vi "test clear jkism string queue in API1.vi"() -> ()   [LabVIEW 2017]
uses:
  user.lib/_NEVSTOP/Communicable State Machine(CSM)/AdvanceAPI/CSM - Revert Arguments-Safe String.vi
  user.lib/_NEVSTOP/Communicable State Machine(CSM)/AdvanceAPI/CSM - Make String Arguments Safe.vi
  user.lib/_NEVSTOP/Communicable State Machine(CSM)/AdvanceAPI/CSM - Break Down Multiple States String.vi
  user.lib/_NEVSTOP/Communicable State Machine(CSM)/AdvanceAPI/CSM - Compact Multiple States.vi
  user.lib/_NEVSTOP/Communicable State Machine(CSM)/AdvanceAPI/CSM - Keywords.vi
  user.lib/_NEVSTOP/Communicable State Machine(CSM)/_Shared/Trim Single-line Text.vi
  user.lib/_NEVSTOP/Communicable State Machine(CSM)/Communicable State Machine.lvlib
panel:
  in  "API: API1 ->| CSM-Module":bool
  in  "API: API1 -@ CSM-Module":bool
  in  "API: API1 -> CSM-Module":bool
  out "State History 2":string
  out "Error Occurred":errorcluster
  out "State History":string
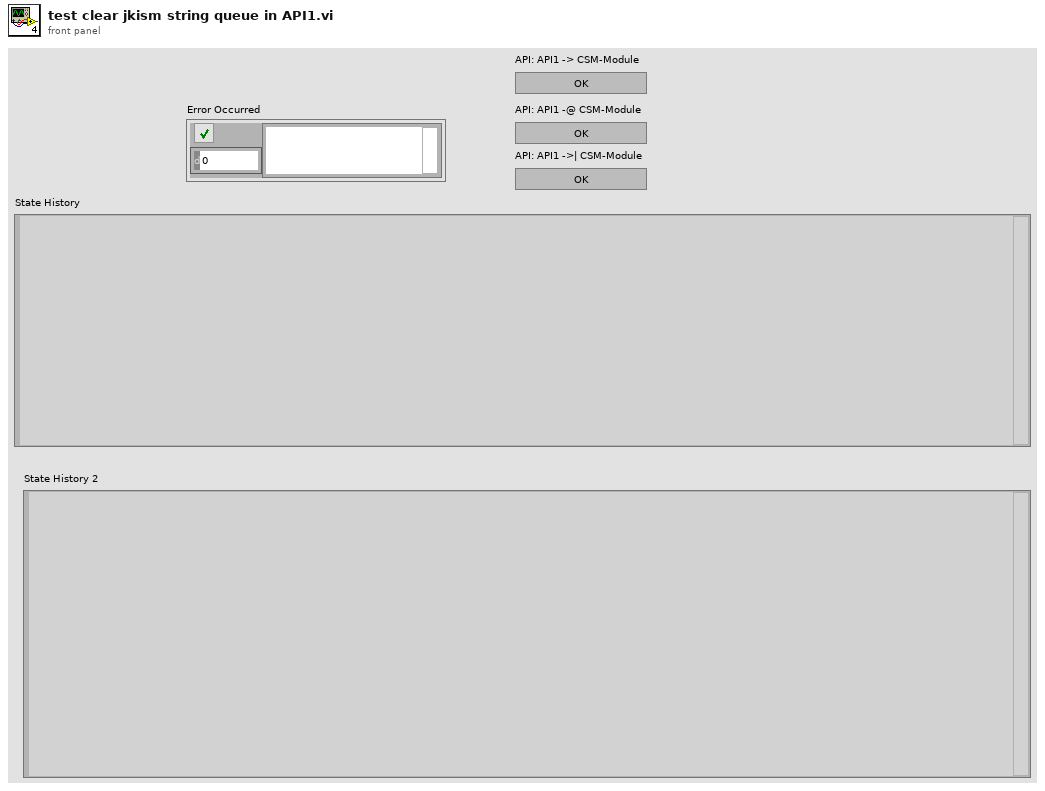
[diagram p1: front panel]
types:
  T1 = enum32{"Invalid", "Standard", "Closed", "Hidden", "Minimized", "Maximized"}
  T2 = enum32{"invalid app kind", "Development System", "Run Time System", "Student Edition", "Embedded LabVIEW", "Evaluation", "Custom"}
  T3 = typedef "Communicable State Machine.lvlib/_CSM_Response Source Message.ctl" = cluster{"‘State":string, "’Arguments":string, "’Error":errorcluster}
  T4 = cluster{"Current VI Reference":refnum<vi>, "Close Panel on Exit?":bool}
  T5 = cluster{"Core":cluster{"Current VI Reference":refnum<vi>, "Close Panel on Exit?":bool}, "Your Boolean data":bool, "Your string data":string}
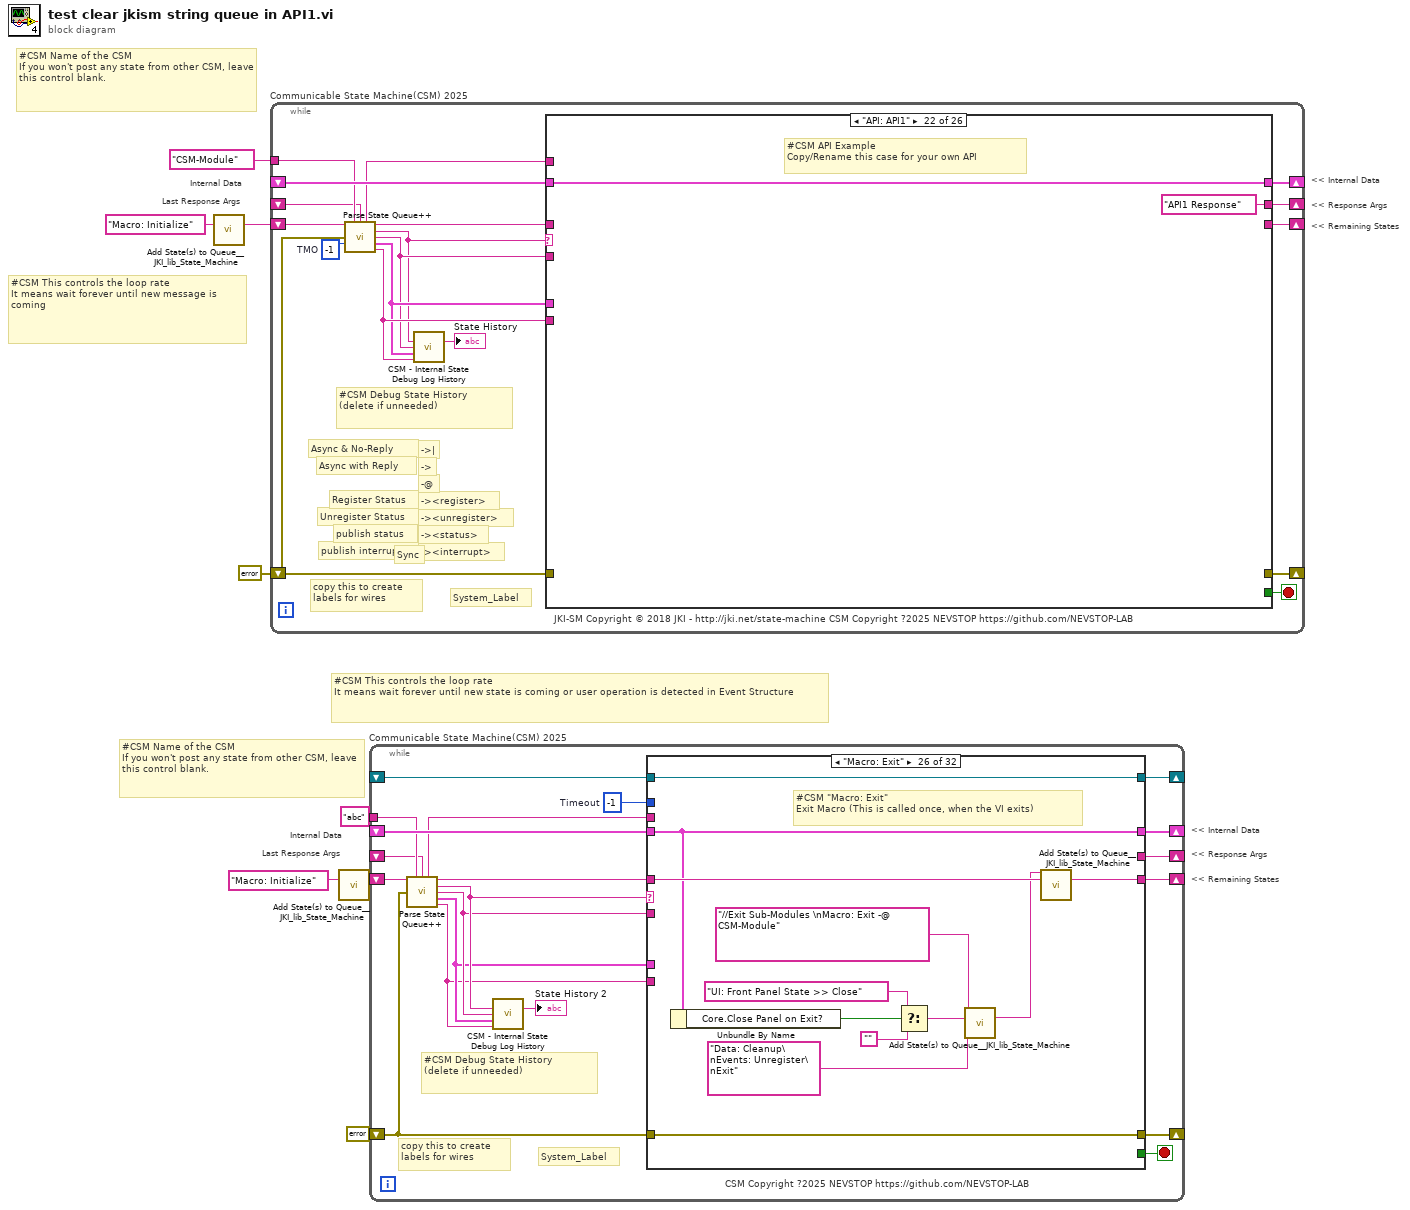
[diagram p0: block diagram]
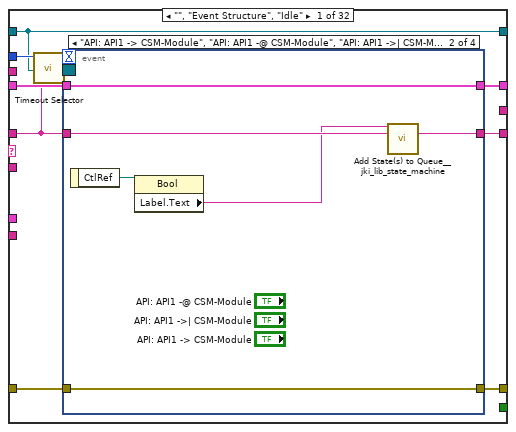
[diagram p2: hidden frame]
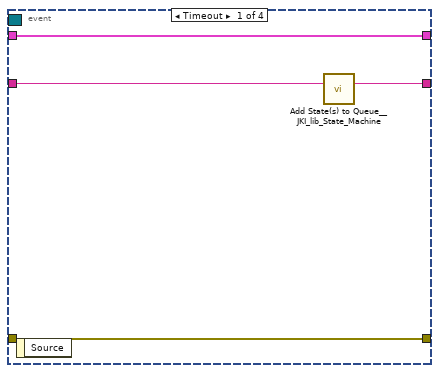
[diagram p3: hidden frame]
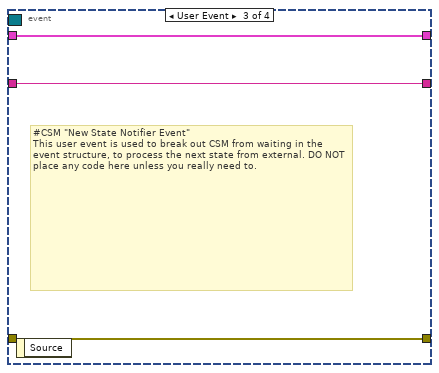
[diagram p4: hidden frame]
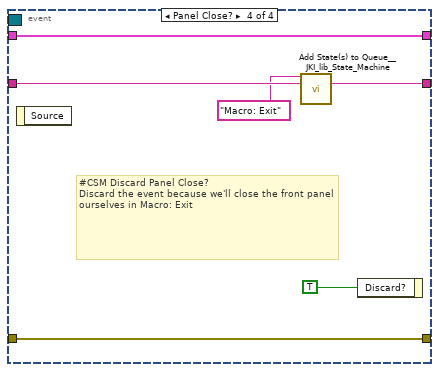
[diagram p5: hidden frame]
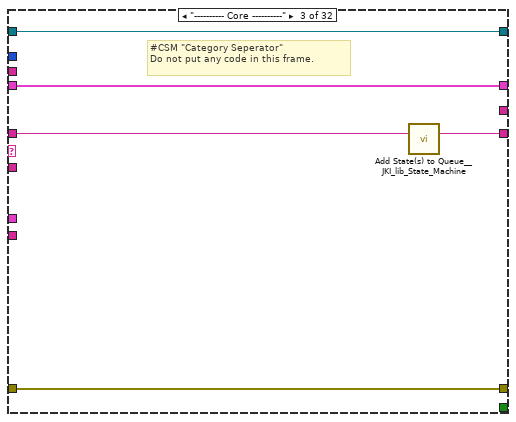
[diagram p7: hidden frame]
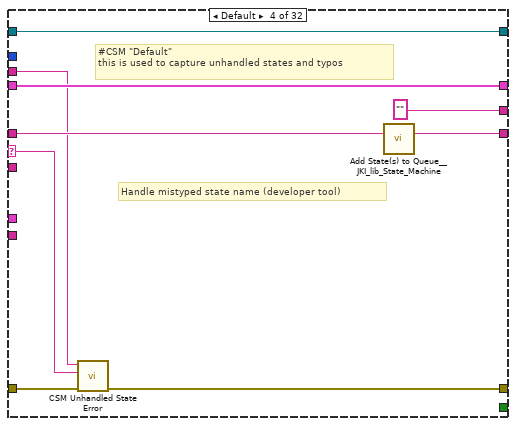
[diagram p8: hidden frame]
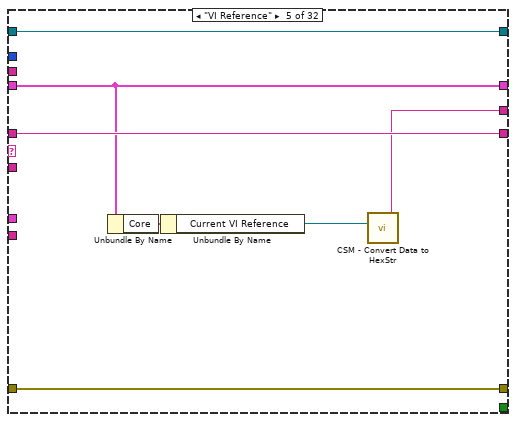
[diagram p9: hidden frame]
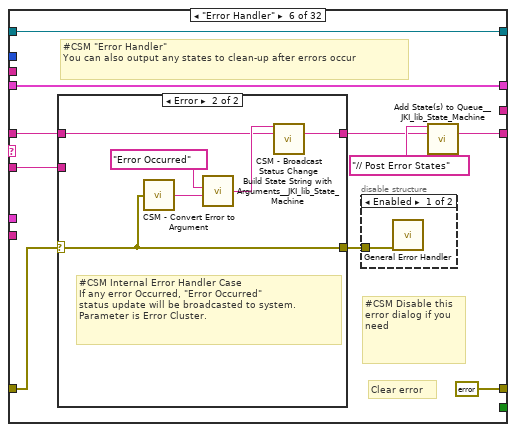
[diagram p10: hidden frame]
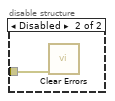
[diagram p11: hidden frame]
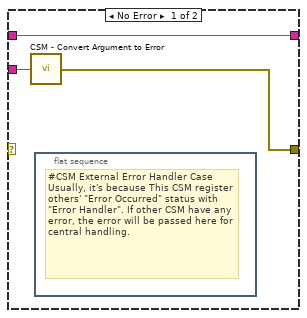
[diagram p12: hidden frame]
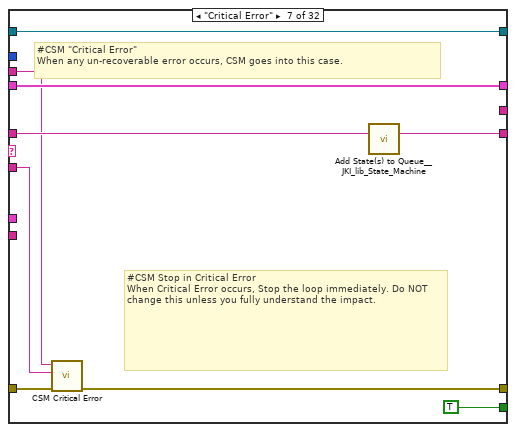
[diagram p13: hidden frame]
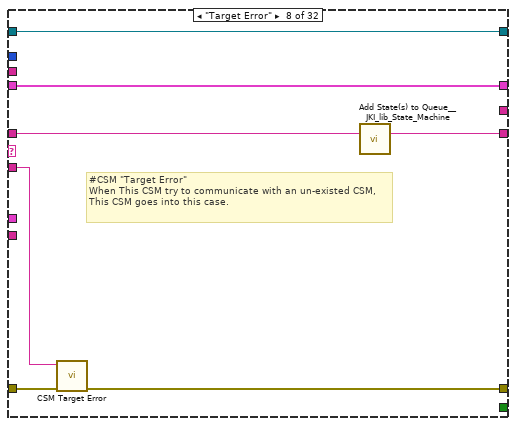
[diagram p14: hidden frame]
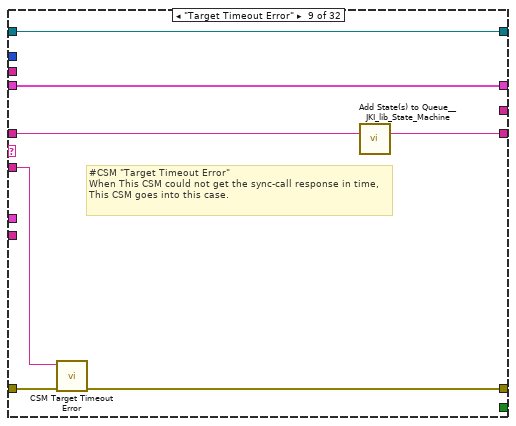
[diagram p15: hidden frame]
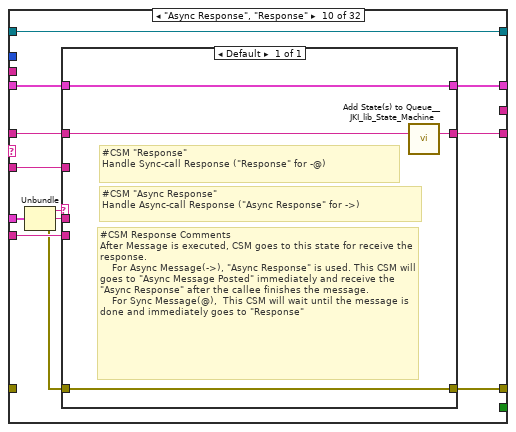
[diagram p16: hidden frame]
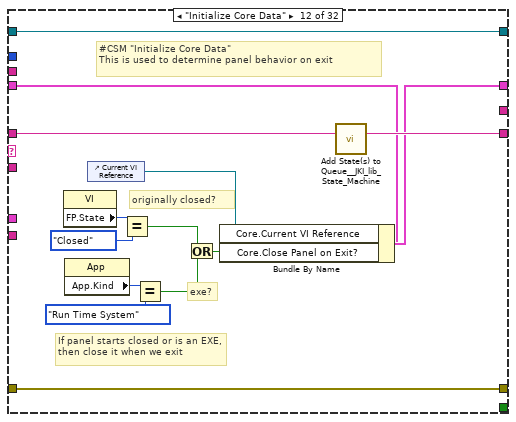
[diagram p18: hidden frame]
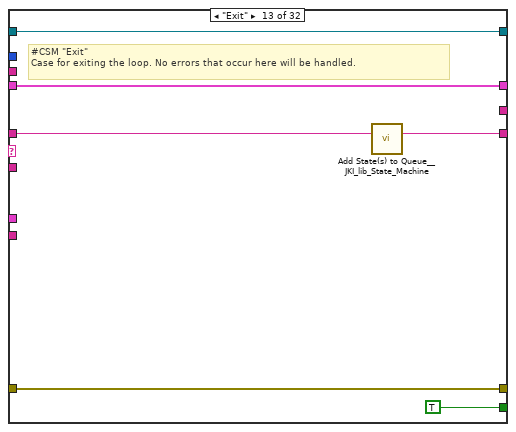
[diagram p19: hidden frame]
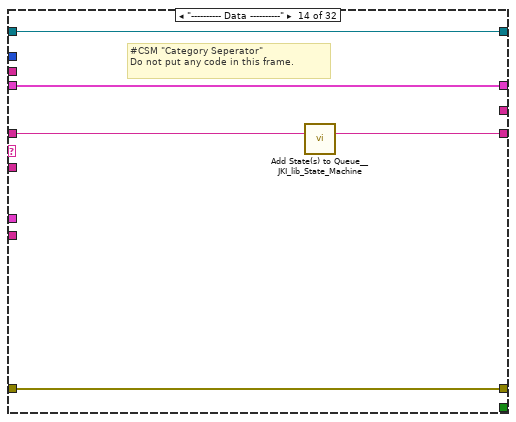
[diagram p20: hidden frame]
diagram:
  # "Last Response Args"
  # "Internal Data"
  # "#CSM Name of the CSM\nIf you won't post any state from other CSM, leave this control blank."
  # "#CSM This controls the loop rate\nIt means wait forever until new state is coming or user operation is detected in Event Structure"
  # "<< Internal Data"
  # "<< Response Args"
  # "<< Remaining States"
  # "Last Response Args"
  # "Internal Data"
  # "#CSM Name of the CSM\nIf you won't post any state from other CSM, leave this control blank."
  # "#CSM This controls the loop rate\nIt means wait forever until new message is coming"
  # "<< Internal Data"
  # "<< Response Args"
  # "<< Remaining States"
  n1 = call <vilib>:"Add State(s) to Queue__JKI_lib_State_Machine.vi"("State(s) in (\"\")"="Macro: Initialize" ("Init State(\"Macro: Initialize\")")) -> ("States Out"=w5:string)  [unwired: 14 in]
  n2 = while "Communicable State Machine(CSM) 2025" {
    shift-right: [w21] -> _
    shift-left: _ -> [w20]
    shift-right: [w24] -> _
    shift-left: errorcluster {"status"=FALSE, "code"=0, "source"=""} ("error out") -> [w10]
    shift-right: [w23] -> _
    shift-left: w5 -> [w25]
    tunnel: "CSM-Module" ("Name (\"\" to Use UUID)") -> [w17]
    shift-right: [w18] -> _
    shift-left: _ -> [w12]
    stop <- w22 stop-if-true
    w19 = -1  # TMO
    # "#CSM Debug State History\n(delete if unneeded)"
    # "-><interrupt>"
    # "-><status>"
    # "-><unregister>"
    # "-><register>"
    # "-@"
    # "->"
    # "->|"
    # "publish interrupt"
    # "publish status"
    # "Unregister Status"
    # "Register Status"
    # "Sync"
    # "Async with Reply"
    # "Async & No-Reply"
    # "JKI-SM Copyright © 2018 JKI - http://jki.net/state-machine CSM Copyright ?2025 NEVSTOP https://github.com/NEVSTOP-LAB"
    # "copy this to create labels for wires"
    # "System_Label"
    n3 = call "Parse State Queue++.vi"("State Queue"=w25, "Name (\"\" to Use UUID)"=w17, "Response Arguments"=w12, "Previous Error"=w10, "Dequeue (1 ms)"=w19) -> ("Name Used"=w11:string, "Remaining States"=w26:string, "Current State"=w13:string, "Arguments"=w14:string, "Additional Information"=w15:T3, "Source CSM"=w16:string)  [unwired: 5 in]
    n4 = call "CSM - Internal State Debug Log History.vi"("State"=w13, "Arguments (\"\")"=w14, ">> Response Source Message >>"=w15, "Source (\"\")"=w16) -> ("Debug Log"=→"State History":string)  [unwired: 11 in]
    n5 = case shown="\"API: API1\"" w13 {
      selector: w13 -> [_ _ _ w37 _ _ _ _ _ _ _ _ _ _ _ _ _ _ _ _ _ _ _ _ _ _]
      tunnel: w26 -> [w27 w30 w33 w41 w46 w51 w74 w80 w86 w96 w103 w115 w119 w122 w128 w130 w136 w139 w143 w149 w151 _ w157 w162 w165 w168]
      tunnel: w14 -> [_ _ _ _ _ w50 w70 w77 w83 w90 _ _ _ _ _ _ _ _ _ _ _ _ w155 _ _ _]
      tunnel: w20 -> [w28 w29 w31 w39 w45 w56 w72 w78 w84 w94 w102 w109 w117 w120 _ w129 w131 w137 w141 w147 w150 w153 w156 w160 w163 w166]
      tunnel: [_ _ _ w34 w47 errorcluster {"status"=FALSE, "code"=0, "source"=""} ("error out") w67 w75 w81 w97 _ _ _ _ _ _ w132 _ _ _ _ _ _ _ _ _] -> w24
      tunnel: w10 -> [_ _ _ w35 w47 w54 w68 w76 w82 _ _ _ _ _ _ _ w133 _ _ _ _ _ _ _ _ _]
      tunnel: [w27 w30 w32 w40 w46 w52 w73 w79 w85 w95 w103 w114 w118 w121 w127 w130 w135 w138 w142 w148 w151 _ w157 w161 w164 w167] -> w23
      tunnel: [_ _ _ _ _ _ TRUE _ _ _ _ _ TRUE _ _ _ _ _ _ _ _ _ _ _ _ _] -> w22
      tunnel: [w28 w29 w31 w39 w45 w56 w72 w78 w84 w93 w102 w113 w117 w120 w126 w129 w131 w137 w141 w147 w150 w153 w156 w160 w163 w166] -> w21
      tunnel: w16 -> [_ _ _ _ _ w49 _ _ _ w91 _ _ _ _ _ _ _ _ _ _ _ _ _ _ _ _]
      tunnel: w15 -> [_ _ _ _ _ w48 _ _ _ w92 _ _ _ _ _ _ _ _ _ _ _ _ _ _ _ _]
      tunnel: [_ _ _ "" w42 _ _ _ _ _ _ _ _ _ _ _ _ _ _ _ _ "API1 Response" w154 _ _ _] -> w18
      tunnel: w11 -> [_ _ _ w36 _ _ w69 _ _ _ _ _ _ _ _ _ _ _ _ _ _ _ _ _ _ _]
      frame "", "Idle" {
        # "#CSM \"Idle/Event Handler\"\nexecutes when the state queue is empty"
      }
      frame "CSM Documentation" {
        # "#CSM State Syntax\n\n// Comment line, all text to the right of “//” will be ignored\n// Local Message Example\nDoSth: DoA >> Arguments\n\n// Sync Call Example\nAPI: xxxx >> Arguments -@ TargetModule\n\n// Async Call Example\nAPI: xxxx >> Arguments -> TargetModule\n\n// Async Call without Reply Example\nAPI: xxxx >> Arguments ->| TargetModule\n\n// Broadcast normal status:\nStatus >> StatusArguments  -><status>\n\n// Broadcast Interrupt status:\nInterrupt >> StatusArguments  -><interrupt>\n\n// Register Source Module's status to Handler Module\nStatus@Source Module >> Handler Module@Handler Module -><register>\n\n// Unegister Source Module's status\nStatus@Source Module >> Handler Module -><unregister>"
        # "#CSM README FIRST\n\nCommunicable State Machine(CSM) is a LabVIEW application framework that builds upon JKI State Machine(JKISM). It follows the pattern of JKISM and extends the keywords to describe message communication between modules, including concepts such as Sync-Message, Async-Message, Subscription/Unsubscription of status - essential elements for creating reusable code modules. For more information, please visit the CSM wiki: https://nevstop-lab.github.io/CSM-Wiki/\n\nFor instructions on JKI State Machine, visit: \n    http://jki.net/state-machine/\nFor information about CSM, visit: \n    https://github.com/NEVSTOP-LAB"
        # "#CSM \"Documentation\"\nCase for holding CSM Documenation"
      }
      frame "---------- Core ----------" {
        # "#CSM \"Category Seperator\"\nDo not put any code in this frame."
        n6 = call <vilib>:"Add State(s) to Queue__JKI_lib_State_Machine.vi"("State(s) in (\"\")"=w33) -> ("States Out"=w32:string)  [unwired: 14 in]
      }
      frame Default {
        # "#CSM \"Default\"\nthis is used to capture unhandled states and typos"
        n7 = call "CSM Unhandled State Error.vi"("error in (no error)"=w35, "Undefined State"=w37, "CSM Name"=w36) -> ("error out"=w34:errorcluster)  [unwired: 8 in]
        n8 = call <vilib>:"Add State(s) to Queue__JKI_lib_State_Machine.vi"("State(s) in (\"\")"=w41) -> ("States Out"=w40:string)  [unwired: 14 in]
      }
      frame "VI Reference" {
        n9 = Unbundle By Name(w45) -> ("Core"=w44:T4)
        n10 = Unbundle By Name(w44) -> ("Current VI Reference"=w43:refnum<vi>)
        n11 = call "CSM - Convert Data to HexStr.vi"("Variant"=w43) -> ("HEX String (0-9,A-F)"=w42:string)  [unwired: 8 in]
      }
      frame "Error Handler" {
        # "#CSM \"Error Handler\"\nYou can also output any states to clean-up after errors occur"
        # "Clear error"
        n12 = case shown="No Error" w54 {
          selector: w54 -> [_ w61]
          tunnel: [w60 w63] -> w53
          tunnel: w51 -> [w60 w62]
          tunnel: w50 -> [w59 _]
          tunnel: w49 -> [_ _]
          tunnel: w48 -> [_ _]
          frame No Error {
            n13 = call "CSM - Convert Argument to Error.vi"("Argument"=w59) -> ("Error"=w58:errorcluster)  [unwired: 4 in]
            n14 = flat-sequence {
              tunnel: w58 -> [_]
              frame #0 {
                # "#CSM External Error Handler Case\nUsually, it's because This CSM register others' \"Error Occurred\" status with \"Error Handler\". If other CSM have any error, the error will be passed here for central handling."
              }
            }
          }
          frame Error {
            # "#CSM Internal Error Handler Case \nIf any error Occurred, \"Error Occurred\" \nstatus update will be broadcasted to system.\nParameter is Error Cluster."
            n15 = call "CSM - Convert Error to Argument.vi"("Error"=w61) -> ("Argument"=w65:string)  [unwired: 4 in]
            n16 = call <vilib>:"Build State String with Arguments__JKI_lib_State_Machine.vi"("Arguments (\"\")"=w65, "State"="Error Occurred" ("Status with Arguments")) -> ("State with Arguments"=w64:string)  [unwired: 4 in]
            n17 = call "CSM - Broadcast Status Change.vi"("Status With Arguments"=w64, "State Queue"=w62) -> ("Remaining States"=w63:string)  [unwired: 13 in]
            "Error Occurred" <- w61
          }
        }
        n18 = call <vilib>:"Add State(s) to Queue__JKI_lib_State_Machine.vi"("State(s) in Front (\"\")"="// Post Error States", "State(s) in (\"\")"=w53) -> ("States Out"=w52:string)  [unwired: 13 in]
      }
      frame "Critical Error" {
        # "#CSM \"Critical Error\"\nWhen any un-recoverable error occurs, CSM goes into this case."
        # "#CSM Stop in Critical Error\nWhen Critical Error occurs, Stop the loop immediately. Do NOT change this unless you fully understand the impact."
        n19 = call "CSM Critical Error.vi"("error in (no error)"=w68, "Arugments (As Reason)"=w70, "CSM Name"=w69) -> ("error out"=w67:errorcluster)  [unwired: 8 in]
        n20 = call <vilib>:"Add State(s) to Queue__JKI_lib_State_Machine.vi"("State(s) in (\"\")"=w74) -> ("States Out"=w73:string)  [unwired: 14 in]
      }
      frame "Target Timeout Error" {
        # "#CSM \"Target Timeout Error\"\nWhen This CSM could not get the sync-call response in time, This CSM goes into this case."
        n21 = call "CSM Target Timeout Error.vi"("error in (no error)"=w76, "Arguments (As CSM Name)"=w77) -> ("error out"=w75:errorcluster)  [unwired: 9 in]
        n22 = call <vilib>:"Add State(s) to Queue__JKI_lib_State_Machine.vi"("State(s) in (\"\")"=w80) -> ("States Out"=w79:string)  [unwired: 14 in]
      }
      frame "Target Error" {
        # "#CSM \"Target Error\"\nWhen This CSM try to communicate with an un-existed CSM, This CSM goes into this case."
        n23 = call "CSM Target Error.vi"("error in (no error)"=w82, "Arguments (As CSM Name)"=w83) -> ("error out"=w81:errorcluster)  [unwired: 9 in]
        n24 = call <vilib>:"Add State(s) to Queue__JKI_lib_State_Machine.vi"("State(s) in (\"\")"=w86) -> ("States Out"=w85:string)  [unwired: 14 in]
      }
      frame "Async Response", "Response" {
        n25 = Unbundle(w92) -> ("‘State"=w89:string, "’Arguments"=w88:string, "’Error"=w87:errorcluster)
        n26 = case shown="Default" w89 {
          tunnel: [w98] -> w95
          tunnel: w96 -> [w99]
          tunnel: [w101] -> w93
          tunnel: w94 -> [w101]
          tunnel: [w100] -> w97
          tunnel: w87 -> [w100]
          tunnel: w91 -> [_]
          tunnel: w90 -> [_]
          tunnel: w88 -> [_]
          frame Default {
            # "#CSM \"Async Response\"\nHandle Async-call Response (\"Async Response\" for ->)"
            # "#CSM \"Response\"\nHandle Sync-call Response (\"Response\" for -@)"
            # "#CSM Response Comments\nAfter Message is executed, CSM goes to this state for receive the response.\n    For Async Message(->), \"Async Response\" is used. This CSM will goes to \"Async Message Posted\" immediately and receive the \"Async Response\" after the callee finishes the message.\n    For Sync Message(@),  This CSM will wait until the message is done and immediately goes to \"Response\""
            n27 = call <vilib>:"Add State(s) to Queue__JKI_lib_State_Machine.vi"("State(s) in (\"\")"=w99) -> ("States Out"=w98:string)  [unwired: 14 in]
          }
        }
      }
      frame "Async Message Posted" {
        # "#CSM \"Async Message Posted\"\nAfter Async Message is posted (-> or ->| ), CSM goes to this state for post-action.\nYou can use Argument - State to tell which Async Message is called."
      }
      frame "Initialize Core Data" {
        # "#CSM \"Initialize Core Data\"\nThis is used to determine panel behavior on exit"
        # "originally closed?"
        # "exe?"
        # "If panel starts closed or is an EXE, then close it when we exit"
        n28 = control-ref of="Current VI Reference"() -> (w107:refnum<vi>)
        n29 = property class="VI"() -> ("FP.State"=w106:T1)  [unwired: 2 in, 2 out]
        n30 = property class="App"() -> ("App.Kind"=w112:T2)  [unwired: 2 in, 2 out]
        n31 = Equal?(x=w106, y=T1."Closed" ("Front Panel Window:State")) -> (x = y?=w104:bool)
        n32 = Equal?(x=w112, y=T2."Run Time System" ("Application:Kind")) -> (x = y?=w110:bool)
        n33 = Or(x=w104, y=w110) -> (x .or. y?=w108:bool)
        n34 = Bundle By Name(cluster=w109, "Core.Current VI Reference"=w107, "Core.Close Panel on Exit?"=w108) -> (w113:T5)
        n35 = call <vilib>:"Add State(s) to Queue__JKI_lib_State_Machine.vi"("State(s) in (\"\")"=w115) -> ("States Out"=w114:string)  [unwired: 14 in]
      }
      frame "Exit" {
        # "#CSM \"Exit\"\nCase for exiting the loop. No errors that occur here will be handled."
        n36 = call <vilib>:"Add State(s) to Queue__JKI_lib_State_Machine.vi"("State(s) in (\"\")"=w119) -> ("States Out"=w118:string)  [unwired: 14 in]
      }
      frame "---------- Data ----------" {
        # "#CSM \"Category Seperator\"\nDo not put any code in this frame."
        n37 = call <vilib>:"Add State(s) to Queue__JKI_lib_State_Machine.vi"("State(s) in (\"\")"=w122) -> ("States Out"=w121:string)  [unwired: 14 in]
      }
      frame "Data: Initialize" {
        w123 = T4 {"Current VI Reference"=refnum, "Close Panel on Exit?"=FALSE}  # Core
        w125 = TRUE  # Your Boolean data
        w124 = ""  # Your string data
        # "#CSM \"Data: Initialize\"\nInitialize the shift-register data, here.\n(data names are defined by what you wire into the bundle function)"
        # "#CSM do not delete - used by framework"
        # "#CSM Expand Bundle to add new data elements to shift register data."
        # "#CSM Add new data here."
        # "#CSM Data names and types of shift register data are defined by this bundle."
        n38 = Bundle("Core"=w123, "Your Boolean data"=w125, "Your string data"=w124) -> (w126:T5)  [unwired: 1 in]
        n39 = call <vilib>:"Add State(s) to Queue__JKI_lib_State_Machine.vi"("State(s) in (\"\")"=w128) -> ("States Out"=w127:string)  [unwired: 14 in]
      }
      frame "Data: Update Indicators" {
      }
      frame "Data: Cleanup" {
        # "#CSM \"Data: Cleanup\"\nCleanup any data and references, here.\n(this is called automatically, by the Macro: Exit)"
        n40 = Unbundle By Name(w131) -> ("Core.Current VI Reference"=w134:refnum<vi>)
        n41 = Close Reference(reference=w134, error in (no error)=w133) -> (error out=w132:errorcluster)
        n42 = call <vilib>:"Add State(s) to Queue__JKI_lib_State_Machine.vi"("State(s) in (\"\")"=w136) -> ("States Out"=w135:string)  [unwired: 14 in]
      }
      frame "---------- Macro ----------" {
        # "#CSM \"Category Seperator\"\nDo not put any code in this frame."
        n43 = call <vilib>:"Add State(s) to Queue__JKI_lib_State_Machine.vi"("State(s) in (\"\")"=w139) -> ("States Out"=w138:string)  [unwired: 14 in]
      }
      frame "Macro: Initialize" {
        # "#CSM \"Macro: Initialize\"\nInitialization Macro (This is called once, when the VI starts)"
        n44 = call <vilib>:"Add State(s) to Queue__JKI_lib_State_Machine.vi"("State(s) in Front (\"\")"="Data: Initialize\nInitialize Core Data\nData: Update Indicators", "State(s) in (\"\")"=w143) -> ("States Out"=w142:string)  [unwired: 13 in]
      }
      frame "Macro: Exit" {
        # "#CSM \"Macro: Exit\"\nExit Macro (This is called once, when the VI exits)"
        n45 = call <vilib>:"Add State(s) to Queue__JKI_lib_State_Machine.vi"("State(s) in Front (\"\")"="//Exit Sub-Modules ", "State(s) at Back (\"\")"="Data: Cleanup\nExit") -> ("States Out"=w145:string)  [unwired: 13 in]
        n46 = call <vilib>:"Add State(s) to Queue__JKI_lib_State_Machine.vi"("State(s) in Front (\"\")"=w145, "State(s) in (\"\")"=w149) -> ("States Out"=w148:string)  [unwired: 13 in]
      }
      frame "---------- API ----------" {
        # "#CSM \"Category Seperator\"\nDo not put any code in this frame."
      }
      frame "API: API1" {
        # "#CSM API Example\nCopy/Rename this case for your own API"
      }
      frame "API: API2" {
        # "#CSM API Example\nCopy/Rename this case for your own API"
        # "unpack Hex String  to Variant\nif complex parameter is needed."
        n47 = call "CSM - Convert HexStr to Data.vi"("HEX String"=w155) -> ()  [unwired: 7 in, 2 out]
        n48 = disable-structure shown="Disabled" {
          disable-tunnel: [w158 "API2 Response"] -> w154
          frame Disabled {
            # "pack variant to hexstr \nif complex response is needed."
            # "complex Response"
            n49 = call "CSM - Convert Data to HexStr.vi"() -> ("HEX String (0-9,A-F)"=w158:string)  [unwired: 9 in]
          }
          frame Enabled {
          }
        }
      }
      frame "---------- Action ----------" {
        # "#CSM \"Category Seperator\"\nDo not put any code in this frame."
        n50 = call <vilib>:"Add State(s) to Queue__JKI_lib_State_Machine.vi"("State(s) in (\"\")"=w162) -> ("States Out"=w161:string)  [unwired: 14 in]
      }
      frame "Action: action1" {
        # "#CSM \"Internal State\"\nThis category is used for holding internal states"
        n51 = call <vilib>:"Add State(s) to Queue__JKI_lib_State_Machine.vi"("State(s) in (\"\")"=w165) -> ("States Out"=w164:string)  [unwired: 14 in]
      }
      frame "Action: action2" {
        # "#CSM \"Internal State\"\nThis category is used for holding internal states"
        n52 = call <vilib>:"Add State(s) to Queue__JKI_lib_State_Machine.vi"("State(s) in (\"\")"=w168) -> ("States Out"=w167:string)  [unwired: 14 in]
      }
    }
  }
  n53 = call <vilib>:"Add State(s) to Queue__JKI_lib_State_Machine.vi"("State(s) in (\"\")"="Macro: Initialize" ("Init State(\"Macro: Initialize\")")) -> ("States Out"=w1:string)  [unwired: 14 in]
  n54 = while "Communicable State Machine(CSM) 2025" {
    shift-right: [w183] -> _
    shift-left: _ -> [w182]
    shift-right: [w186] -> _
    shift-left: errorcluster {"status"=FALSE, "code"=0, "source"=""} ("error out") -> [w180]
    shift-right: [w185] -> _
    shift-left: w1 -> [w187]
    tunnel: "abc" ("Name (\"\" to Use UUID) 2") -> [w176]
    shift-right: [w179] -> _
    shift-left: _ -> [w170]
    shift-right: [w178] -> _
    shift-left: _ -> [w177]
    stop <- w184 stop-if-true
    w181 = -1  # Timeout
    # "#CSM Debug State History\n(delete if unneeded)"
    # "copy this to create labels for wires"
    # "System_Label"
    # "CSM Copyright ?2025 NEVSTOP https://github.com/NEVSTOP-LAB"
    n55 = call "Parse State Queue++.vi"("State Queue"=w187, "Name (\"\" to Use UUID)"=w176, "Response Arguments"=w170, "Previous Error"=w180) -> ("Name Used"=w171:string, "Remaining States"=w188:string, "Current State"=w175:string, "Arguments"=w174:string, "Additional Information"=w173:T3, "Source CSM"=w172:string)  [unwired: 6 in]
    n56 = call "CSM - Internal State Debug Log History.vi"("State"=w175, "Arguments (\"\")"=w174, ">> Response Source Message >>"=w173, "Source (\"\")"=w172) -> ("Debug Log"=→"State History 2":string)  [unwired: 11 in]
    n57 = case shown="\"Macro: Exit\"" w175 {
      selector: w175 -> [_ _ _ w228 _ _ _ _ _ _ _ _ _ _ _ _ _ _ _ _ _ _ _ _ _ _ _ _ _ _ _ _]
      tunnel: w188 -> [w189 w219 w225 w233 w240 w246 w269 w275 w282 w291 w304 w319 w325 w330 w338 w345 w350 w357 w361 w367 w372 w379 w395 w465 w471 w483 w486 w491 w497 w505 w510 w515]
      tunnel: w174 -> [_ _ _ _ _ w245 w264 w274 w281 w290 _ _ _ _ _ _ _ _ _ _ _ w374 w389 _ _ _ _ _ w494 _ _ _]
      tunnel: w182 -> [w196 w218 w222 w231 w239 w250 w270 w277 w284 w293 w303 w312 w323 w327 _ w340 w347 w356 w360 w364 w370 w377 w391 w462 w468 w480 w485 w490 w496 w502 w507 w512]
      tunnel: [w195 w220 w223 w226 w241 errorcluster {"status"=FALSE, "code"=0, "source"=""} ("error out") w265 w272 w279 w296 w305 w316 w322 w328 w335 w341 w348 w351 w359 w365 w369 w375 w392 w463 w469 w481 w487 w492 w498 w503 w508 w513] -> w186
      tunnel: w180 -> [w194 w220 w223 w234 w241 w247 w271 w273 w280 _ w305 w316 w322 w328 w335 w342 w348 _ w362 w365 w369 w376 w393 w463 w469 w481 w487 w492 w498 w503 w508 w513]
      tunnel: [w197 w219 w224 w232 w240 w242 w268 w278 w285 w292 w304 w318 w324 w329 w337 w344 w349 w357 w361 w366 w371 w378 w394 w464 w470 w482 w486 w491 w497 w504 w509 w514] -> w185
      tunnel: [_ _ _ _ _ _ TRUE _ _ _ _ _ TRUE _ _ _ _ _ _ _ _ _ _ _ _ _ _ _ _ _ _ _] -> w184
      tunnel: [w193 w218 w222 w231 w239 w250 w270 w277 w284 w294 w303 w317 w323 w327 w336 w340 w347 w356 w360 w364 w370 w377 w391 w462 w468 w480 w485 w490 w496 w502 w507 w512] -> w183
      tunnel: w181 -> [w192 _ _ _ _ _ _ _ _ _ _ _ _ _ _ _ _ _ _ _ _ _ _ _ _ _ _ _ _ _ _ _]
      tunnel: w172 -> [_ _ _ _ _ _ _ _ _ w288 _ _ _ _ _ _ _ _ _ _ _ _ _ _ _ _ _ _ _ _ _ _]
      tunnel: w173 -> [_ _ _ _ _ _ _ _ _ w295 _ _ _ _ _ _ _ _ _ _ _ _ _ _ _ _ _ _ _ _ _ _]
      tunnel: [_ _ _ "" w235 _ _ _ _ _ _ _ _ _ _ _ _ _ _ _ _ _ _ _ _ _ _ "API1 Response" w493 _ _ _] -> w179
      tunnel: [w191 w217 w221 w229 w238 w249 w266 w276 w283 w297 w302 w306 w320 w326 w331 w339 w346 w355 w358 w363 w368 w373 w388 w461 w466 w473 w484 w489 w495 w501 w506 w511] -> w178
      tunnel: w177 -> [w191 w217 w221 w229 w238 w249 w266 w276 w283 w297 w302 w306 w320 w326 w331 w339 w346 _ w358 w363 w368 w373 w388 w461 w466 w473 w484 w489 w495 w501 w506 w511]
      tunnel: w171 -> [_ _ _ w227 _ _ w263 _ _ _ _ _ _ _ _ _ _ w354 _ _ _ _ _ _ _ _ _ _ _ _ _ _]
      frame "", "Event Structure", "Idle" {
        n58 = call "Timeout Selector.vi"("Remaining States"=w189, "Timeout Expected"=w192) -> ("Timeout"=w190:i32)  [unwired: 5 in]
        n59 = event shown="[1] \"API: API1 -> CSM-Module\", \"API: API1 -@ CSM-Module\", \"API: API1 ->| CSM-Module\": Value Change" {
          selector: w191 -> [_ _ _ _]
          dyn-events: _ -> [_ _ _ _]
          timeout: w190 -> [_ _ _ _]
          tunnel: w189 -> [w201 w203 w209 w216]
          tunnel: [w200 w204 w209 w215] -> w197
          tunnel: w196 -> [w198 w206 w210 w213]
          tunnel: [w199 w207 w208 w214] -> w195
          tunnel: w194 -> [w199 w207 w208 w214]
          tunnel: [w198 w206 w210 w213] -> w193
          event Timeout {
            n60 = event-data() -> ()  [unwired: 1 in, 1 out]
            n61 = call <vilib>:"Add State(s) to Queue__JKI_lib_State_Machine.vi"("State(s) in (\"\")"=w201) -> ("States Out"=w200:string)  [unwired: 14 in]
          }
          event "API: API1 -> CSM-Module", "API: API1 -@ CSM-Module", "API: API1 ->| CSM-Module": Value Change {
            n62 = event-data() -> ("CtlRef"=w205:refnum<vi>)  [unwired: 1 in]
            n63 = property class="Bool"(reference=w205) -> ("Label.Text"=w202:string)  [unwired: 1 in, 2 out]
            n64 = call <vilib>:"Add State(s) to Queue__jki_lib_state_machine.vi"("State(s) in Front (\"\")"=w202, "State(s) in (\"\")"=w203) -> ("States Out"=w204:string)  [unwired: 13 in]
          }
          event User Event {
            # "#CSM \"New State Notifier Event\"\nThis user event is used to break out CSM from waiting in the event structure, to process the next state from external. DO NOT place any code here unless you really need to."
            n65 = event-data() -> ()  [unwired: 1 in, 1 out]
          }
          event Panel Close? {
            # "#CSM Discard Panel Close?\nDiscard the event because we'll close the front panel ourselves in Macro: Exit"
            n66 = event-data() -> ()  [unwired: 1 in, 1 out]
            n67 = call <vilib>:"Add State(s) to Queue__JKI_lib_State_Machine.vi"("State(s) in Front (\"\")"="Macro: Exit", "State(s) in (\"\")"=w216) -> ("States Out"=w215:string)  [unwired: 13 in]
            n68 = event-data("Discard?"=TRUE) -> ()  [unwired: 1 in, 1 out]
          }
        }
      }
      frame "CSM Documentation" {
        # "#CSM README FIRST\n\nCommunicable State Machine(CSM) is a LabVIEW application framework that builds upon JKI State Machine(JKISM). It follows the pattern of JKISM and extends the keywords to describe message communication between modules, including concepts such as Sync-Message, Async-Message, Subscription/Unsubscription of status - essential elements for creating reusable code modules. For more information, please visit the CSM wiki: https://nevstop-lab.github.io/CSM-Wiki/\n\nFor instructions on JKI State Machine, visit: http://jki.net/state-machine/\nFor information about CSM, visit: https://github.com/NEVSTOP-LAB"
        # "#CSM \"Documentation\"\nCase for holding CSM Documenation"
      }
      frame "---------- Core ----------" {
        # "#CSM \"Category Seperator\"\nDo not put any code in this frame."
        n69 = call <vilib>:"Add State(s) to Queue__JKI_lib_State_Machine.vi"("State(s) in (\"\")"=w225) -> ("States Out"=w224:string)  [unwired: 14 in]
      }
      frame Default {
        # "#CSM \"Default\"\nthis is used to capture unhandled states and typos"
        # "Handle mistyped state name (developer tool)"
        n70 = call "CSM Unhandled State Error.vi"("error in (no error)"=w234, "Undefined State"=w228, "CSM Name"=w227) -> ("error out"=w226:errorcluster)  [unwired: 8 in]
        n71 = call <vilib>:"Add State(s) to Queue__JKI_lib_State_Machine.vi"("State(s) in (\"\")"=w233) -> ("States Out"=w232:string)  [unwired: 14 in]
      }
      frame "VI Reference" {
        n72 = Unbundle By Name(w239) -> ("Core"=w237:T4)
        n73 = Unbundle By Name(w237) -> ("Current VI Reference"=w236:refnum<vi>)
        n74 = call "CSM - Convert Data to HexStr.vi"("Variant"=w236) -> ("HEX String (0-9,A-F)"=w235:string)  [unwired: 8 in]
      }
      frame "Error Handler" {
        # "#CSM Disable this error dialog if you need"
        # "#CSM \"Error Handler\"\nYou can also output any states to clean-up after errors occur"
        # "Clear error"
        n75 = case shown="Error" w247 {
          selector: w247 -> [_ w257]
          tunnel: [w256 w259] -> w243
          tunnel: w246 -> [w256 w258]
          tunnel: w245 -> [w255 _]
          tunnel: [w254 w257] -> w248
          frame No Error {
            n76 = call "CSM - Convert Argument to Error.vi"("Argument"=w255) -> ("Error"=w254:errorcluster)  [unwired: 4 in]
            n77 = flat-sequence {
              frame #0 {
                # "#CSM External Error Handler Case\nUsually, it's because This CSM register others' \"Error Occurred\" status with \"Error Handler\". If other CSM have any error, the error will be passed here for central handling."
              }
            }
          }
          frame Error {
            # "#CSM Internal Error Handler Case \nIf any error Occurred, \"Error Occurred\" \nstatus update will be broadcasted to system.\nParameter is Error Cluster."
            n78 = call "CSM - Convert Error to Argument.vi"("Error"=w257) -> ("Argument"=w261:string)  [unwired: 4 in]
            n79 = call <vilib>:"Build State String with Arguments__JKI_lib_State_Machine.vi"("Arguments (\"\")"=w261, "State"="Error Occurred" ("Status with Arguments")) -> ("State with Arguments"=w260:string)  [unwired: 4 in]
            n80 = call "CSM - Broadcast Status Change.vi"("Status With Arguments"=w260, "State Queue"=w258) -> ("Remaining States"=w259:string)  [unwired: 13 in]
          }
        }
        n81 = disable-structure shown="Enabled" {
          disable-tunnel: w248 -> [w252 w253]
          frame Enabled {
            n82 = call <vilib>:"General Error Handler.vi"("error in (no error)"=w252) -> ()  [unwired: 10 in, 5 out]
          }
          frame Disabled {
            n83 = call <vilib>:"Clear Errors.vi"("error in (no error)"=w253) -> ()  [unwired: 5 in, 2 out]
          }
        }
        n84 = call <vilib>:"Add State(s) to Queue__JKI_lib_State_Machine.vi"("State(s) in Front (\"\")"="// Post Error States", "State(s) in (\"\")"=w243) -> ("States Out"=w242:string)  [unwired: 13 in]
      }
      frame "Critical Error" {
        # "#CSM Stop in Critical Error\nWhen Critical Error occurs, Stop the loop immediately. Do NOT change this unless you fully understand the impact."
        # "#CSM \"Critical Error\"\nWhen any un-recoverable error occurs, CSM goes into this case."
        n85 = call "CSM Critical Error.vi"("error in (no error)"=w271, "Arugments (As Reason)"=w264, "CSM Name"=w263) -> ("error out"=w265:errorcluster)  [unwired: 8 in]
        n86 = call <vilib>:"Add State(s) to Queue__JKI_lib_State_Machine.vi"("State(s) in (\"\")"=w269) -> ("States Out"=w268:string)  [unwired: 14 in]
      }
      frame "Target Error" {
        # "#CSM \"Target Error\"\nWhen This CSM try to communicate with an un-existed CSM, This CSM goes into this case."
        n87 = call "CSM Target Error.vi"("error in (no error)"=w273, "Arguments (As CSM Name)"=w274) -> ("error out"=w272:errorcluster)  [unwired: 9 in]
        n88 = call <vilib>:"Add State(s) to Queue__JKI_lib_State_Machine.vi"("State(s) in (\"\")"=w275) -> ("States Out"=w278:string)  [unwired: 14 in]
      }
      frame "Target Timeout Error" {
        # "#CSM \"Target Timeout Error\"\nWhen This CSM could not get the sync-call response in time, This CSM goes into this case."
        n89 = call "CSM Target Timeout Error.vi"("error in (no error)"=w280, "Arguments (As CSM Name)"=w281) -> ("error out"=w279:errorcluster)  [unwired: 9 in]
        n90 = call <vilib>:"Add State(s) to Queue__JKI_lib_State_Machine.vi"("State(s) in (\"\")"=w282) -> ("States Out"=w285:string)  [unwired: 14 in]
      }
      frame "Async Response", "Response" {
        n91 = Unbundle(w295) -> ("‘State"=w289:string, "’Arguments"=w287:string, "’Error"=w286:errorcluster)
        n92 = case shown="Default" w289 {
          tunnel: [w301] -> w296
          tunnel: w286 -> [w301]
          tunnel: [w300] -> w294
          tunnel: w293 -> [w300]
          tunnel: [w298] -> w292
          tunnel: w291 -> [w299]
          tunnel: w290 -> [_]
          tunnel: w288 -> [_]
          tunnel: w287 -> [_]
          frame Default {
            # "#CSM Response Comments\nAfter Message is executed, CSM goes to this state for receive the response.\n    For Async Message(->), \"Async Response\" is used. This CSM will goes to \"Async Message Posted\" immediately and receive the \"Async Response\" after the callee finishes the message.\n    For Sync Message(@),  This CSM will wait until the message is done and immediately goes to \"Response\""
            # "#CSM \"Async Response\"\nHandle Async-call Response (\"Async Response\" for ->)"
            # "#CSM \"Response\"\nHandle Sync-call Response (\"Response\" for -@)"
            n93 = call <vilib>:"Add State(s) to Queue__JKI_lib_State_Machine.vi"("State(s) in (\"\")"=w299) -> ("States Out"=w298:string)  [unwired: 14 in]
          }
        }
      }
      frame "Async Message Posted" {
        # "#CSM \"Async Message Posted\"\nAfter Async Message is posted (-> or ->| ), CSM goes to this state for post-action.\nYou can use Argument - State to tell which Async Message is called."
      }
      frame "Initialize Core Data" {
        # "#CSM \"Initialize Core Data\"\nThis is used to determine panel behavior on exit"
        # "originally closed?"
        # "exe?"
        # "If panel starts closed or is an EXE, then close it when we exit"
        n94 = property class="VI"() -> ("FP.State"=w309:T1)  [unwired: 2 in, 2 out]
        n95 = property class="App"() -> ("App.Kind"=w315:T2)  [unwired: 2 in, 2 out]
        n96 = control-ref of="Current VI Reference"() -> (w310:refnum<vi>)
        n97 = Equal?(x=w309, y=T1."Closed" ("Front Panel Window:State")) -> (x = y?=w307:bool)
        n98 = Equal?(x=w315, y=T2."Run Time System" ("Application:Kind")) -> (x = y?=w313:bool)
        n99 = Or(x=w307, y=w313) -> (x .or. y?=w311:bool)
        n100 = Bundle By Name(cluster=w312, "Core.Current VI Reference"=w310, "Core.Close Panel on Exit?"=w311) -> (w317:T5)
        n101 = call <vilib>:"Add State(s) to Queue__JKI_lib_State_Machine.vi"("State(s) in (\"\")"=w319) -> ("States Out"=w318:string)  [unwired: 14 in]
      }
      frame "Exit" {
        # "#CSM \"Exit\"\nCase for exiting the loop. No errors that occur here will be handled."
        n102 = call <vilib>:"Add State(s) to Queue__JKI_lib_State_Machine.vi"("State(s) in (\"\")"=w325) -> ("States Out"=w324:string)  [unwired: 14 in]
      }
      frame "---------- Data ----------" {
        # "#CSM \"Category Seperator\"\nDo not put any code in this frame."
        n103 = call <vilib>:"Add State(s) to Queue__JKI_lib_State_Machine.vi"("State(s) in (\"\")"=w330) -> ("States Out"=w329:string)  [unwired: 14 in]
      }
      frame "Data: Initialize" {
        w332 = T4 {"Current VI Reference"=refnum, "Close Panel on Exit?"=FALSE}  # Core
        w334 = TRUE  # Your Boolean data
        w333 = ""  # Your string data
        # "#CSM do not delete - used by framework"
        # "#CSM Expand Bundle to add new data elements to shift register data."
        # "#CSM Add new data here."
        # "Initialize the shift-register data, here.\n(data names are defined by what you wire into the bundle function)"
        n104 = Bundle("Core"=w332, "Your Boolean data"=w334, "Your string data"=w333) -> (w336:T5)  [unwired: 1 in]
        n105 = call <vilib>:"Add State(s) to Queue__JKI_lib_State_Machine.vi"("State(s) in (\"\")"=w338) -> ("States Out"=w337:string)  [unwired: 14 in]
      }
      frame "Data: Cleanup" {
        # "Cleanup any data and references, here.\n(this is called automatically, by the Macro: Exit)"
        n106 = Unbundle By Name(w340) -> ("Core.Current VI Reference"=w343:refnum<vi>)
        n107 = Close Reference(reference=w343, error in (no error)=w342) -> (error out=w341:errorcluster)
        n108 = call <vilib>:"Add State(s) to Queue__JKI_lib_State_Machine.vi"("State(s) in (\"\")"=w345) -> ("States Out"=w344:string)  [unwired: 14 in]
      }
      frame "---------- Events ----------" {
        # "#CSM \"Category Seperator\"\nDo not put any code in this frame."
        n109 = call <vilib>:"Add State(s) to Queue__JKI_lib_State_Machine.vi"("State(s) in (\"\")"=w350) -> ("States Out"=w349:string)  [unwired: 14 in]
      }
      frame "Events: Register" {
        # "#CSM \"Events: Register\"\nRegister user event. New Message Event is registered to break CSM waiting in event structure by default."
        # "#CSM Register New Message Event\nRegister message event to break Waiting in Event structure."
        n110 = call "CSM - Get New State Notifier Event.vi"("Name (\"\" to Use UUID)"=w354) -> ("error out"=w352:errorcluster, "New State Notifier Event"=w353:refnum<user-event>)  [unwired: 9 in]
        n111 = register-events(error in=w352, w353) -> (reference out=w355:refnum<event-registration>, error out=w351:errorcluster)  [unwired: 1 in]
      }
      frame "Events: Unregister" {
        # "#CSM \"Events: Unregister\"\nUnregister user event."
        n112 = Unregister For Events(event registration refnum=w358, error in=w362) -> (error out=w359:errorcluster)
      }
      frame "---------- UI ----------" {
        # "#CSM \"Category Seperator\"\nDo not put any code in this frame."
        n113 = call <vilib>:"Add State(s) to Queue__JKI_lib_State_Machine.vi"("State(s) in (\"\")"=w367) -> ("States Out"=w366:string)  [unwired: 14 in]
      }
      frame "UI: Initialize" {
        # "#CSM \"UI: Initialize\"\nInitialize the User Interface, here.\n(this is called automatically, by the Macro: Init)"
        n114 = call <vilib>:"Add State(s) to Queue__JKI_lib_State_Machine.vi"("State(s) in (\"\")"=w372) -> ("States Out"=w371:string)  [unwired: 14 in]
      }
      frame "UI: Cursor Set" {
        # "#CSM \"UI: Cursor Set\"\nSet and Unset Cursor Busy.\n(Usage: \"UI: Cursor Set >> Busy|Idle\")"
        # "Argument"
        n115 = disable-structure shown="Default" {
          disable-tunnel: w376 -> [w382 w387]
          disable-tunnel: [w381 w387] -> w375
          disable-tunnel: w374 -> [w380 _]
          frame condition #0 (active) {
            n116 = case shown="\"Idle\", Default" w380 {
              tunnel: w382 -> [w384 w386]
              tunnel: [w383 w385] -> w381
              frame "Idle", Default {
                n117 = call <vilib>:"Unset Busy.vi"("error in (no error)"=w384) -> ("error out"=w383:errorcluster)  [unwired: 10 in]
              }
              frame "Busy" {
                n118 = call <vilib>:"Set Busy.vi"("error in (no error)"=w386) -> ("error out"=w385:errorcluster)  [unwired: 9 in, 1 out]
              }
            }
          }
          frame condition #1 {
          }
        }
        n119 = call <vilib>:"Add State(s) to Queue__JKI_lib_State_Machine.vi"("State(s) in (\"\")"=w379) -> ("States Out"=w378:string)  [unwired: 14 in]
      }
      frame "UI: Front Panel State" {
        # "#CSM \"UI: Front Panel State\"\nSet Front Panel Open or Closed\n(Usage: \"UI: Front Panel State >> Open|Close\")"
        # "Argument"
        n120 = Unbundle By Name(w391) -> ("Core.Current VI Reference"=w390:refnum<vi>)
        n121 = call <vilib>:"Add State(s) to Queue__JKI_lib_State_Machine.vi"("State(s) in (\"\")"=w395) -> ("States Out"=w394:string)  [unwired: 14 in]
        n122 = case shown="\"Close\", \"Closed\"" w389 {
          tunnel: w393 -> [w401 w416 w427 w440 w453]
          tunnel: [w403 w417 w429 w442 w455] -> w392
          tunnel: w390 -> [w402 w414 w428 w441 w454]
          frame "Open", "Standard", Default {
            w396 = T1."Standard" ("State")
            n123 = property class="VI"(reference=w402, error in=w401) -> (reference out=w399:refnum<vi>, error out=w400:errorcluster, "FP.State"=w398:T1)
            n124 = Not Equal?(x=w398, y=w396) -> (x != y?=w397:bool)
            n125 = case shown="True" w397 {
              tunnel: [w407 w409] -> w403
              tunnel: w400 -> [w406 w409]
              tunnel: w399 -> [w405 _]
              tunnel: w396 -> [w404 _]
              frame True {
                n126 = invoke class="VI" method="FP.Open"(reference=w405, error in=w406, "Activate"=TRUE, "State"=w404) -> (error out=w407:errorcluster)  [unwired: 1 in, 4 out]
              }
              frame False {
              }
            }
          }
          frame "Close", "Closed" {
            n127 = property class="VI"(reference=w414, error in=w416) -> (reference out=w413:refnum<vi>, error out=w415:errorcluster, "FP.State"=w411:T1)
            n128 = Not Equal?(x=w411, y=T1."Closed" ("Front Panel Window:State")) -> (x != y?=w410:bool)
            n129 = case shown="False" w410 {
              tunnel: [w418 w421] -> w417
              tunnel: w415 -> [w418 w420]
              tunnel: w413 -> [_ w419]
              frame False {
              }
              frame True {
                n130 = invoke class="VI" method="FP.Close"(reference=w419, error in=w420) -> (error out=w421:errorcluster)  [unwired: 1 in, 2 out]
              }
            }
          }
          frame "Hidden", "Hide" {
            w422 = T1."Hidden" ("State")
            n131 = property class="VI"(reference=w428, error in=w427) -> (reference out=w425:refnum<vi>, error out=w426:errorcluster, "FP.State"=w424:T1)
            n132 = Not Equal?(x=w424, y=w422) -> (x != y?=w423:bool)
            n133 = case shown="True" w423 {
              tunnel: [w433 w434] -> w429
              tunnel: w426 -> [w432 w434]
              tunnel: w425 -> [w431 _]
              tunnel: w422 -> [w430 _]
              frame True {
                n134 = invoke class="VI" method="FP.Open"(reference=w431, error in=w432, "State"=w430) -> (error out=w433:errorcluster)  [unwired: 2 in, 4 out]
              }
              frame False {
              }
            }
          }
          frame "Minimize", "Minimized" {
            w435 = T1."Minimized" ("State")
            n135 = property class="VI"(reference=w441, error in=w440) -> (reference out=w438:refnum<vi>, error out=w439:errorcluster, "FP.State"=w437:T1)
            n136 = Not Equal?(x=w437, y=w435) -> (x != y?=w436:bool)
            n137 = case shown="True" w436 {
              tunnel: [w446 w447] -> w442
              tunnel: w439 -> [w445 w447]
              tunnel: w438 -> [w444 _]
              tunnel: w435 -> [w443 _]
              frame True {
                n138 = invoke class="VI" method="FP.Open"(reference=w444, error in=w445, "State"=w443) -> (error out=w446:errorcluster)  [unwired: 2 in, 4 out]
              }
              frame False {
              }
            }
          }
          frame "Maximize", "Maximized" {
            w448 = T1."Maximized" ("State")
            n139 = property class="VI"(reference=w454, error in=w453) -> (reference out=w451:refnum<vi>, error out=w452:errorcluster, "FP.State"=w450:T1)
            n140 = Not Equal?(x=w450, y=w448) -> (x != y?=w449:bool)
            n141 = case shown="True" w449 {
              tunnel: [w459 w460] -> w455
              tunnel: w452 -> [w458 w460]
              tunnel: w451 -> [w457 _]
              tunnel: w448 -> [w456 _]
              frame True {
                n142 = invoke class="VI" method="FP.Open"(reference=w457, error in=w458, "State"=w456) -> (error out=w459:errorcluster)  [unwired: 2 in, 4 out]
              }
              frame False {
              }
            }
          }
        }
      }
      frame "---------- Macro ----------" {
        # "#CSM \"Category Seperator\"\nDo not put any code in this frame."
        n143 = call <vilib>:"Add State(s) to Queue__JKI_lib_State_Machine.vi"("State(s) in (\"\")"=w465) -> ("States Out"=w464:string)  [unwired: 14 in]
      }
      frame "Macro: Initialize" {
        w467 = "Data: Initialize\nInitialize Core Data\nEvents: Register\nUI: Initialize\nUI: Front Panel State >> Open"  # Data: Initialize Initialize Core Data Events: Register UI: Initialize UI: Front Panel State >> Open
        # "#CSM \"Macro: Initialize\"\nInitialization Macro (This is called once, when the VI starts)"
        n144 = call <vilib>:"Add State(s) to Queue__JKI_lib_State_Machine.vi"("State(s) in Front (\"\")"=w467, "State(s) in (\"\")"=w471) -> ("States Out"=w470:string)  [unwired: 13 in]
      }
      frame "Macro: Exit" {
        # "#CSM \"Macro: Exit\"\nExit Macro (This is called once, when the VI exits)"
        n145 = Unbundle By Name(w480) -> ("Core.Close Panel on Exit?"=w479:bool)
        n146 = Select(t="UI: Front Panel State >> Close", s=w479, f="") -> (s? t:f=w476:string)
        n147 = call <vilib>:"Add State(s) to Queue__JKI_lib_State_Machine.vi"("State(s) in Front (\"\")"="//Exit Sub-Modules \nMacro: Exit -@ CSM-Module", "State(s) in (\"\")"=w476, "State(s) at Back (\"\")"="Data: Cleanup\nEvents: Unregister\nExit") -> ("States Out"=w474:string)  [unwired: 12 in]
        n148 = call <vilib>:"Add State(s) to Queue__JKI_lib_State_Machine.vi"("State(s) in Front (\"\")"=w474, "State(s) in (\"\")"=w483) -> ("States Out"=w482:string)  [unwired: 13 in]
      }
      frame "---------- API ----------" {
        # "#CSM \"Category Seperator\"\nDo not put any code in this frame."
      }
      frame "API: API1" {
        # "#CSM API Example\nCopy/Rename this case for your own API"
        # "#CSM Response\nConnect this to return the response of your API"
        # "#CSM >> Source CSM >>\nIf you need to tell who triggered this state , use this string. If it's this case itself, this string is \"\"."
        # "#CSM >> Arguments >>\nDeal with the parameter if any"
      }
      frame "API: API2" {
        # "#CSM API Example\nCopy/Rename this case for your own API"
        # "unpack Hex String  to Variant\nif complex parameter is needed."
        n149 = call "CSM - Convert HexStr to Data.vi"("HEX String"=w494) -> ()  [unwired: 7 in, 2 out]
        n150 = disable-structure shown="Disabled" {
          disable-tunnel: [w499 "API2 Response"] -> w493
          frame Disabled {
            # "pack variant to hexstr \nif complex response is needed."
            # "complex Response"
            n151 = call "CSM - Convert Data to HexStr.vi"() -> ("HEX String (0-9,A-F)"=w499:string)  [unwired: 9 in]
          }
          frame Enabled {
          }
        }
      }
      frame "---------- Action ----------" {
        # "#CSM \"Category Seperator\"\nDo not put any code in this frame."
        n152 = call <vilib>:"Add State(s) to Queue__JKI_lib_State_Machine.vi"("State(s) in (\"\")"=w505) -> ("States Out"=w504:string)  [unwired: 14 in]
      }
      frame "Action: action1" {
        # "#CSM \"Internal State\"\nThis category is used for holding internal states"
        n153 = call <vilib>:"Add State(s) to Queue__JKI_lib_State_Machine.vi"("State(s) in (\"\")"=w510) -> ("States Out"=w509:string)  [unwired: 14 in]
      }
      frame "Action: action2" {
        # "#CSM \"Internal State\"\nThis category is used for holding internal states"
        n154 = call <vilib>:"Add State(s) to Queue__JKI_lib_State_Machine.vi"("State(s) in (\"\")"=w515) -> ("States Out"=w514:string)  [unwired: 14 in]
      }
    }
  }
